vi "testing_cw_sweep_multifold_4ch.vi"() -> ()   [LabVIEW 2015, in "Tausand AB1000.lvlib"]
uses:
  <instrlib>/Tausand AB1000/Tausand AB1000.lvlib
  <instrlib>/Tausand AB1000/Public/Controls/counters4ch.ctl
  <instrlib>/Tausand AB1000/Public/Controls/configMultipleCoincRing.ctl
  <instrlib>/Tausand AB1000/Public/Controls/deviceTypeRing.ctl
  <instrlib>/Tausand AB1000/Public/Controls/channelRing.ctl
panel:
  out "device type":T1 items=["any"=0, "AB1002"=1002, "AB1004"=1004, "AB1502"=1502, "AB1504"=1504, "AB2002"=2002, "AB2004"=2004, "AB2502"=2502, "AB2504"=2504]
  out "multifold case":T2[](array[typedef])=[240, 224, 208, 176, 112] items=["ABC"=224, "ABD"=208, "ABE"=200, "ABF"=196, "ABG"=194, "ABH"=193, "ACD"=176, "ACE"=168, "ACF"=164, "ACG"=162, "ACH"=161, "ADE"=152, "ADF"=148, "ADG"=146, "ADH"=145, "AEF"=140, "AEG"=138, "AEH"=137, "AFG"=134, "AFH"=133, "AGH"=131, "BCD"=112, "BCE"=104, "BCF"=100, "BCG"=98, "BCH"=97, "BDE"=88, "BDF"=84, "BDG"=82, "BDH"=81, "BEF"=76, "BEG"=74, "BEH"=73, "BFG"=70, "BFH"=69, "BGH"=67, "CDE"=56, "CDF"=52, "CDG"=50, "CDH"=49, "CEF"=44, "CEG"=42, "CEH"=41, "CFG"=38, "CFH"=37, "CGH"=35, "DEF"=28, "DEG"=26, "DEH"=25, "DFG"=22, "DFH"=21, "DGH"=19, "EFG"=14, "EFH"=13, "EGH"=11, "FGH"=7, "ABCD"=240, "ABCE"=232, "ABCF"=228, "ABCG"=226, "ABCH"=225, "ABDE"=216, "ABDF"=212, "ABDG"=210, "ABDH"=209, "ABEF"=204, "ABEG"=202, "ABEH"=201, "ABFG"=198, "ABFH"=197, "ABGH"=195, "ACDE"=184, "ACDF"=180, "ACDG"=178, "ACDH"=177, "ACEF"=172, "ACEG"=170, "ACEH"=169, "ACFG"=166, "ACFH"=165, "ACGH"=163, "ADEF"=156, "ADEG"=154, "ADEH"=153, "ADFG"=150, "ADFH"=149, "ADGH"=147, "AEFG"=142, "AEFH"=141, "AEGH"=139, "AFGH"=135, "BCDE"=120, "BCDF"=116, "BCDG"=114, "BCDH"=113, "BCEF"=108, "BCEG"=106, "BCEH"=105, "BCFG"=102, "BCFH"=101, "BCGH"=99, "BDEF"=92, "BDEG"=90, "BDEH"=89, "BDFG"=86, "BDFH"=85, "BDGH"=83, "BEFG"=78, "BEFH"=77, "BEGH"=75, "BFGH"=71, "CDEF"=60, "CDEG"=58, "CDEH"=57, "CDFG"=54, "CDFH"=53, "CDGH"=51, "CEFG"=46, "CEFH"=45, "CEGH"=43, "CFGH"=39, "DEFG"=30, "DEFH"=29, "DEGH"=27, "DFGH"=23, "EFGH"=15]
  out "tausand data":u32[][](array[numeric])
  out "current multifold":T2=224 caption="Current multifold" items=["ABC"=224, "ABD"=208, "ABE"=200, "ABF"=196, "ABG"=194, "ABH"=193, "ACD"=176, "ACE"=168, "ACF"=164, "ACG"=162, "ACH"=161, "ADE"=152, "ADF"=148, "ADG"=146, "ADH"=145, "AEF"=140, "AEG"=138, "AEH"=137, "AFG"=134, "AFH"=133, "AGH"=131, "BCD"=112, "BCE"=104, "BCF"=100, "BCG"=98, "BCH"=97, "BDE"=88, "BDF"=84, "BDG"=82, "BDH"=81, "BEF"=76, "BEG"=74, "BEH"=73, "BFG"=70, "BFH"=69, "BGH"=67, "CDE"=56, "CDF"=52, "CDG"=50, "CDH"=49, "CEF"=44, "CEG"=42, "CEH"=41, "CFG"=38, "CFH"=37, "CGH"=35, "DEF"=28, "DEG"=26, "DEH"=25, "DFG"=22, "DFH"=21, "DGH"=19, "EFG"=14, "EFH"=13, "EGH"=11, "FGH"=7, "ABCD"=240, "ABCE"=232, "ABCF"=228, "ABCG"=226, "ABCH"=225, "ABDE"=216, "ABDF"=212, "ABDG"=210, "ABDH"=209, "ABEF"=204, "ABEG"=202, "ABEH"=201, "ABFG"=198, "ABFH"=197, "ABGH"=195, "ACDE"=184, "ACDF"=180, "ACDG"=178, "ACDH"=177, "ACEF"=172, "ACEG"=170, "ACEH"=169, "ACFG"=166, "ACFH"=165, "ACGH"=163, "ADEF"=156, "ADEG"=154, "ADEH"=153, "ADFG"=150, "ADFH"=149, "ADGH"=147, "AEFG"=142, "AEFH"=141, "AEGH"=139, "AFGH"=135, "BCDE"=120, "BCDF"=116, "BCDG"=114, "BCDH"=113, "BCEF"=108, "BCEG"=106, "BCEH"=105, "BCFG"=102, "BCFH"=101, "BCGH"=99, "BDEF"=92, "BDEG"=90, "BDEH"=89, "BDFG"=86, "BDFH"=85, "BDGH"=83, "BEFG"=78, "BEFH"=77, "BEGH"=75, "BFGH"=71, "CDEF"=60, "CDEG"=58, "CDEH"=57, "CDFG"=54, "CDFH"=53, "CDGH"=51, "CEFG"=46, "CEFH"=45, "CEGH"=43, "CFGH"=39, "DEFG"=30, "DEFH"=29, "DEGH"=27, "DFGH"=23, "EFGH"=15]
  out "i case":i32
  out "total cases":i32
  in  "Stop Button":bool
  out "coinc Chart":T3(graph)
  out "current values":T4
  in  "sampling (ms)":u32=100
  out "i delay":i32
  out "cw array":u32[](array[numeric])
  in  "step cw":u32=2
  in  "max cw":u32=120
  in  "min cw":u32=2
  out "current cw (ns)":u32
  in  "VISA resource name":refnum<visa-resource-name>
  # "c.win."
  # "case"
  # "out of"
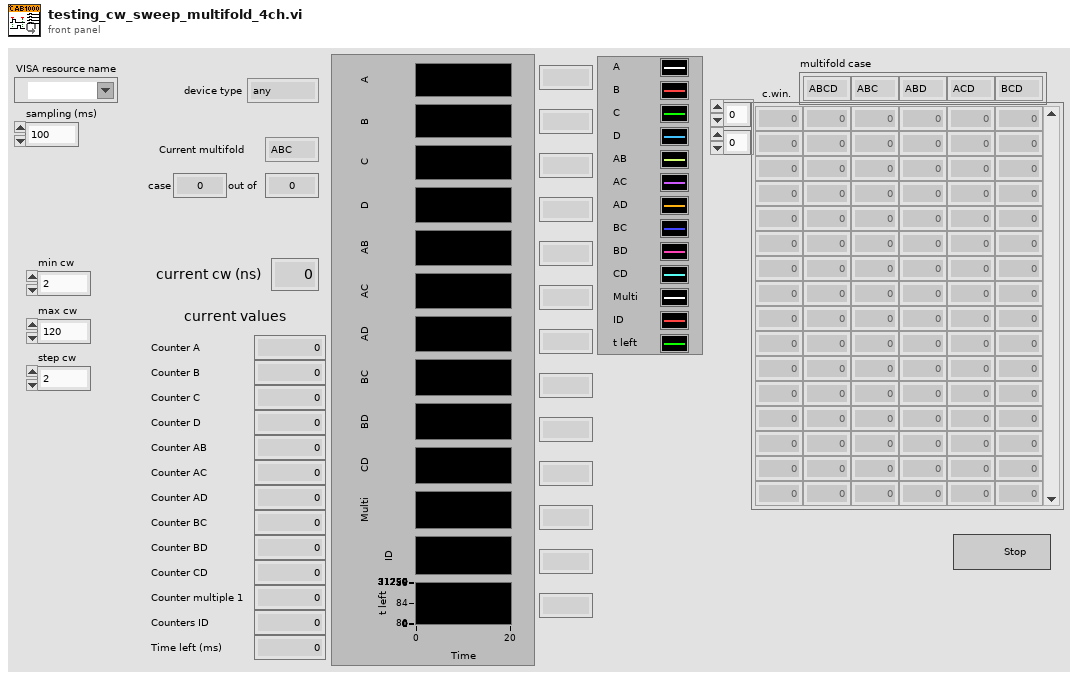
[diagram p1: front panel]
types:
  T1 = typedef "Tausand AB1000.lvlib/deviceTypeRing.ctl" = u16
  T2 = typedef "Tausand AB1000.lvlib/configMultipleCoincRing.ctl" = u16
  T3 = cluster{"counter_A":u32, "counter_B":u32, "counter_C":u32, "counter_D":u32, "counter_AB":u32, "counter_AC":u32, "counter_AD":u32, "counter_BC":u32, "counter_BD":u32, "counter_CD":u32, "counter_multiple_1":u32, "counters_ID":u32, "time_left":u32}
  T4 = typedef "Tausand AB1000.lvlib/counters4ch.ctl" = cluster{"counter_A":u32, "counter_B":u32, "counter_C":u32, "counter_D":u32, "counter_AB":u32, "counter_AC":u32, "counter_AD":u32, "counter_BC":u32, "counter_BD":u32, "counter_CD":u32, "counter_multiple_1":u32, "counters_ID":u32, "time_left":u32}
  T5 = typedef "Tausand AB1000.lvlib/channelRing.ctl" = u8
  T6 = typedef "Tausand AB1000.lvlib/settings4ch.ctl" = cluster{"sampling":u32, "coincidence_window":u32, "delay_A":u32, "delay_B":u32, "delay_C":u32, "delay_D":u32, "sleep_A":u32, "sleep_B":u32, "sleep_C":u32, "sleep_D":u32, "config_multiple_1":T2}
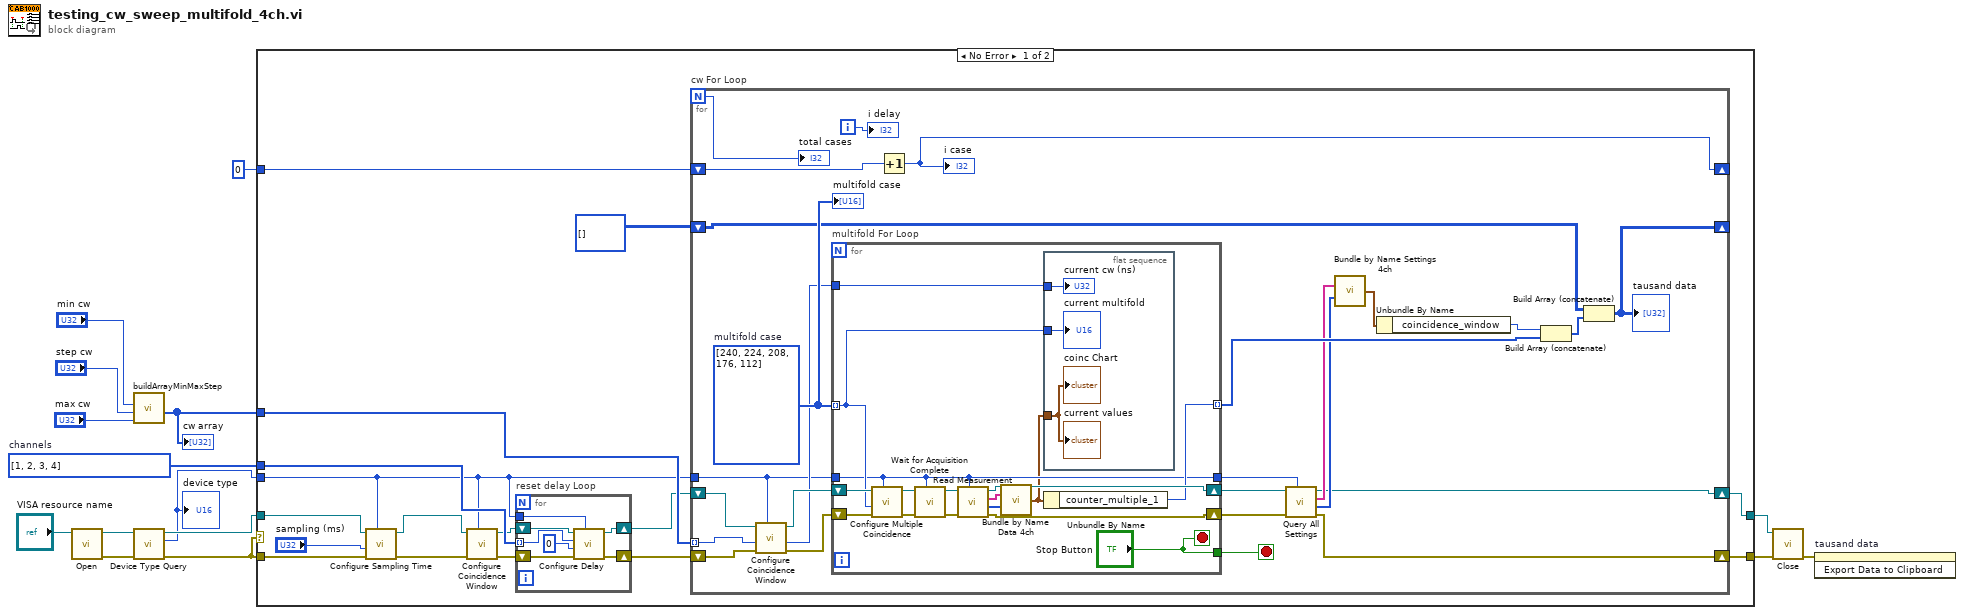
[diagram p0: block diagram]
diagram:
  w6 = T5[] [1, 2, 3, 4] items=["none", "A", "B", "C", "D", "E", "F", "G", "H"]  # channels
  n1 = call <instrlib>:"Open.vi"("VISA resource name"="VISA resource name") -> ("error out"=w11:errorcluster, "VISA resource name out"=w10:refnum<visa-resource-name>)  [unwired: 9 in]
  n2 = call <instrlib>:"buildArrayMinMaxStep.vi"("max (10)"="max cw", "step (1)"="step cw", "min (0)"="min cw") -> ("array"=w7:i32[])  [unwired: 8 in]
  "cw array" <- w7
  n3 = call <instrlib>:"Device Type Query.vi"("error in (no error)"=w11, "VISA Refnum in"=w10) -> ("error out"=w3:errorcluster, "device type"=w8:T1, "VISA Refnum out"=w9:refnum<visa-resource-name>)  [unwired: 7 in]
  "device type" <- w8
  n4 = case shown="No Error" w3 {
    tunnel: w3 -> [w26 w85]
    tunnel: w9 -> [w27 w84]
    tunnel: w8 -> [w25 _]
    tunnel: w7 -> [w31 _]
    tunnel: w6 -> [w28 _]
    tunnel: [w30 w84] -> w5
    tunnel: [w29 w85] -> w4
    tunnel: 0 ("i delay") -> [w21 _]
    frame No Error {
      n5 = call <instrlib>:"Configure Sampling Time.vi"("device type"=w25, "error in (no error)"=w26, "value (1000 ms)"="sampling (ms)", "VISA Refnum in"=w27) -> ("error out"=w23:errorcluster, "VISA Refnum out"=w22:refnum<visa-resource-name>)  [unwired: 5 in, 1 out]
      n6 = call <instrlib>:"Configure Coincidence Window.vi"("device type"=w25, "error in (no error)"=w23, "VISA Refnum in"=w22) -> ("error out"=w19:errorcluster, "VISA Refnum out"=w20:refnum<visa-resource-name>)  [unwired: 6 in, 1 out]
      n7 = for "reset delay Loop" {
        tunnel: w28 -> [w37] mode=indexing
        tunnel: w25 -> [w35]
        shift-right: [w33] -> w17
        shift-left: w19 -> [w34]
        shift-right: [w32] -> w18
        shift-left: w20 -> [w38]
        n8 = call <instrlib>:"Configure Delay.vi"("device type"=w35, "error in (no error)"=w34, "value (0 ns)"=u32 0, "channel"=w37, "VISA Refnum in"=w38) -> ("error out"=w33:errorcluster, "VISA Refnum out"=w32:refnum<visa-resource-name>)  [unwired: 4 in, 1 out]
      }
      n9 = for "cw For Loop" {
        N -> [w59]
        tunnel: w31 -> [w39] mode=indexing
        tunnel: w25 -> [w41]
        shift-right: [w44] -> w29
        shift-left: w17 -> [w63]
        shift-right: [w43] -> w30
        shift-left: w18 -> [w64]
        shift-right: [w60] -> _
        shift-left: w21 -> [w61]
        shift-right: [w52] -> _
        shift-left: u32[][] [] ("tausand data") -> [w54]
        i -> [w62]
        stop <- w42 stop-if-true
        w56 = T2[] [240, 224, 208, 176, 112] items=["ABC"=224, "ABD"=208, "ABE"=200, "ABF"=196, "ABG"=194, "ABH"=193, "ACD"=176, "ACE"=168, "ACF"=164, "ACG"=162, "ACH"=161, "ADE"=152, "ADF"=148, "ADG"=146, "ADH"=145, "AEF"=140, "AEG"=138, "AEH"=137, "AFG"=134, "AFH"=133, "AGH"=131, "BCD"=112, "BCE"=104, "BCF"=100, "BCG"=98, "BCH"=97, "BDE"=88, "BDF"=84, "BDG"=82, "BDH"=81, "BEF"=76, "BEG"=74, "BEH"=73, "BFG"=70, "BFH"=69, "BGH"=67, "CDE"=56, "CDF"=52, "CDG"=50, "CDH"=49, "CEF"=44, "CEG"=42, "CEH"=41, "CFG"=38, "CFH"=37, "CGH"=35, "DEF"=28, "DEG"=26, "DEH"=25, "DFG"=22, "DFH"=21, "DGH"=19, "EFG"=14, "EFH"=13, "EGH"=11, "FGH"=7, "ABCD"=240, "ABCE"=232, "ABCF"=228, "ABCG"=226, "ABCH"=225, "ABDE"=216, "ABDF"=212, "ABDG"=210, "ABDH"=209, "ABEF"=204, "ABEG"=202, "ABEH"=201, "ABFG"=198, "ABFH"=197, "ABGH"=195, "ACDE"=184, "ACDF"=180, "ACDG"=178, "ACDH"=177, "ACEF"=172, "ACEG"=170, "ACEH"=169, "ACFG"=166, "ACFH"=165, "ACGH"=163, "ADEF"=156, "ADEG"=154, "ADEH"=153, "ADFG"=150, "ADFH"=149, "ADGH"=147, "AEFG"=142, "AEFH"=141, "AEGH"=139, "AFGH"=135, "BCDE"=120, "BCDF"=116, "BCDG"=114, "BCDH"=113, "BCEF"=108, "BCEG"=106, "BCEH"=105, "BCFG"=102, "BCFH"=101, "BCGH"=99, "BDEF"=92, "BDEG"=90, "BDEH"=89, "BDFG"=86, "BDFH"=85, "BDGH"=83, "BEFG"=78, "BEFH"=77, "BEGH"=75, "BFGH"=71, "CDEF"=60, "CDEG"=58, "CDEH"=57, "CDFG"=54, "CDFH"=53, "CDGH"=51, "CEFG"=46, "CEFH"=45, "CEGH"=43, "CFGH"=39, "DEFG"=30, "DEFH"=29, "DEGH"=27, "DFGH"=23, "EFGH"=15]  # multifold case
        n10 = call <instrlib>:"Configure Coincidence Window.vi"("device type"=w41, "error in (no error)"=w63, "value ns (10ns)"=w39, "VISA Refnum in"=w64) -> ("error out"=w58:errorcluster, "value ns out"=w51:u32, "VISA Refnum out"=w57:refnum<visa-resource-name>)  [unwired: 5 in]
        n11 = for "multifold For Loop" {
          tunnel: w51 -> [w71]
          tunnel: w41 -> [w66]
          shift-right: [w80] -> w50
          shift-left: w58 -> [w75]
          shift-right: [w79] -> w49
          shift-left: w57 -> [w73]
          tunnel: w56 -> [w70] mode=indexing
          tunnel: [w68] -> w55 mode=indexing
          tunnel: ["Stop Button"] -> w42
          tunnel: [w66] -> w40
          stop <- "Stop Button" stop-if-true
          n12 = call <instrlib>:"Configure Multiple Coincidence.vi"("device type"=w66, "error in (no error)"=w75, "Multiple coincidence configuration"=w70, "VISA Refnum in"=w73) -> ("error out"=w74:errorcluster, "VISA Refnum out"=w72:refnum<visa-resource-name>)  [unwired: 6 in]
          n13 = call <instrlib>:"Wait for Acquisition Complete.vi"("device type"=w66, "error in (no error)"=w74, "VISA resource name"=w72) -> ("error out"=w78:errorcluster, "VISA resource name out"=w77:refnum<visa-resource-name>)  [unwired: 7 in]
          n14 = call <instrlib>:"Read Measurement.vi"("device type"=w66, "error in (no error)"=w78, "VISA Refnum in"=w77) -> ("error out"=w80:errorcluster, "values"=w69:u32[], "labels"=w76:string[], "VISA Refnum out"=w79:refnum<visa-resource-name>)  [unwired: 3 in, 2 out]
          n15 = call <instrlib>:"Bundle by Name Data 4ch.vi"("names"=w76, "values"=w69) -> ("output cluster 4ch"=w65:T4)  [unwired: 13 in]
          n16 = flat-sequence {
            tunnel: w65 -> [w83]
            tunnel: w71 -> [w82]
            tunnel: w70 -> [w81]
            frame #0 {
              "current values" <- w83
              "coinc Chart" <- w83
              "current cw (ns)" <- w82
              "current multifold" <- w81
            }
          }
          n17 = Unbundle By Name(w65) -> ("counter_multiple_1"=w68:u32)
        }
        n18 = Increment(x=w61) -> (x+1=w60:i32)
        "i case" <- w60
        n19 = call <instrlib>:"Query All Settings.vi"("device type"=w40, "error in (no error)"=w50, "VISA Refnum in"=w49) -> ("error out"=w44:errorcluster, "values"=w47:u32[], "labels"=w48:string[], "VISA Refnum out"=w43:refnum<visa-resource-name>)  [unwired: 4 in, 1 out]
        n20 = call <instrlib>:"Bundle by Name Settings 4ch.vi"("names"=w48, "values"=w47) -> ("output cluster settings 4ch"=w46:T6)  [unwired: 13 in]
        n21 = Unbundle By Name(w46) -> ("coincidence_window"=w45:u32)
        n22 = Build Array (concatenate)(w45, w55) -> (w53:u32[])
        n23 = Build Array (concatenate)(w54, w53) -> (w52:u32[][])
        "tausand data" <- w52
        "i delay" <- w62
        "total cases" <- w59
        "multifold case" <- w56
      }
    }
    frame Error {
    }
  }
  n24 = call <instrlib>:"Close.vi"("error in (no error)"=w4, "VISA resource name"=w5) -> ("error out"=w1:errorcluster)  [unwired: 9 in]
  n25 = invoke on="tausand data" class="Arr (strict)" method="Export Data to Clipboard"(error in=w1) -> ()  [unwired: 2 in, 3 out]
